vi "Write_raw_data.vi"(4 "error in":errorcluster, 5 "image_data":u16[][][](array[numeric]), 6 "sequencer":T1(array[cluster]), 7 "ref in":i32) -> (0 "error out":errorcluster, 3 "ref out":i32)   [LabVIEW 2010]
uses:
  <vilib>/addons/h5labview2/dataset/H5Dwrite.llb/H5Dwrite.xnode
  <vilib>/addons/h5labview2/attrib/H5Awrite.llb/H5Awrite.xnode
  <vilib>/addons/h5labview2/base/H5Equery.vi
  <vilib>/addons/h5labview2/group/H5G.lvlib
  <vilib>/addons/h5labview2/h5labview.lib
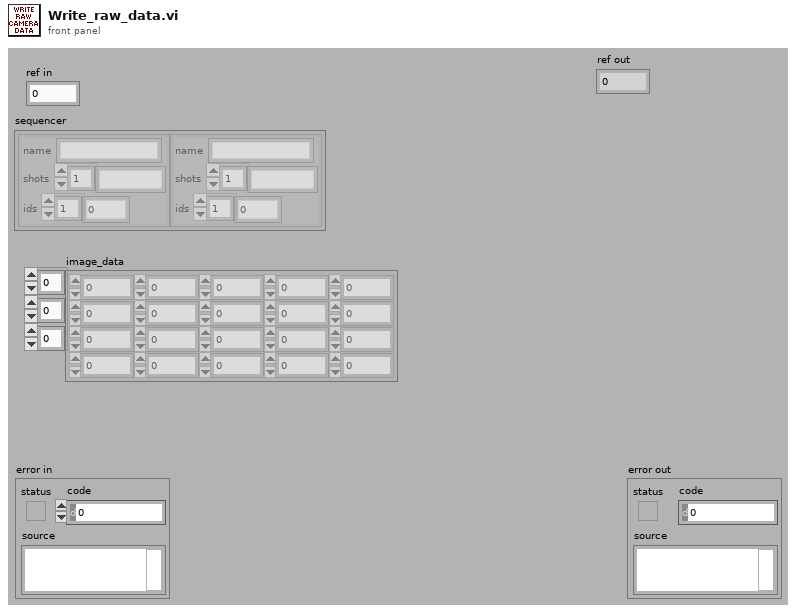
[diagram p1: front panel]
types:
  T1 = cluster{"name":string, "shots":string[], "ids":i32[]}[]
  T2 = typedef "hid_t.ctl" = i32
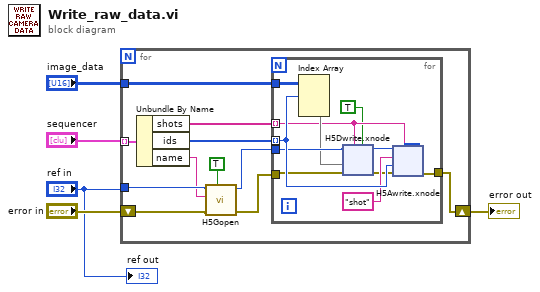
[diagram p0: block diagram]
diagram:
  n1 = for {
    tunnel: "image_data" -> [w16]
    tunnel: "sequencer" -> [w15] mode=indexing
    shift-right: [w12] -> w2
    shift-left: "error in" -> [w9]
    tunnel: "ref in" -> [w8]
    n2 = Unbundle By Name(w15) -> ("shots"=w14:string[], "ids"=w13:i32[], "name"=w7:string)
    n3 = call <vilib>:"H5Gopen.vi"("create? (F)"=TRUE ("Create if not found (F)"), "error in (no error)"=w9, "name"=w7, "ref in"=w8) -> ("error out"=w10:errorcluster, "group out"=w11:T2)  [unwired: 3 in]
    n4 = for {
      tunnel: w10 -> [w20]
      tunnel: w16 -> [w27]
      tunnel: w14 -> [w18] mode=indexing
      tunnel: w13 -> [w25] mode=indexing
      tunnel: [w26] -> w12
      tunnel: w11 -> [w21]
      n5 = Index Array(array=w27, index (dim 0)=w25) -> (element=w19:u16[][])  [unwired: 2 in]
      n6 = xnode "H5Dwrite.xnode"("replace? (F)"=TRUE ("overwrite?"), "dataset name"=w18, "error in (no error)"=w20, "data"=w19, "ref in"=w21) -> ("error out"=w23:errorcluster, "ref out"=w22:i32)  [unwired: 2 in, 1 out]
      n7 = xnode "H5Awrite.xnode"("object name"=w18, "error in (no error)"=w23, "data"=w25, "attrib name"="shot" ("attribute"), "ref in"=w22) -> ("error out"=w26:errorcluster)  [unwired: 2 in, 2 out]
    }
  }
  "error out" <- w2
  "ref out" <- "ref in"
